vi "NiFPGA Read FIFO - Boolean.vi"(6 "Timeout":u32, 8 "error in (no error)":errorcluster, 9 "Number of Elements":u32, 10 "FIFO":u32, 11 "Session":u32) -> (0 "error out":errorcluster, 1 "Data":bool[](array[boolean]), 3 "Session Out":u32, 4 "Elements Remaining":u32)   [LabVIEW 2010, in "FPGA Interface Wrapper.lvlib"]
doc: "Reads from a FIFO of booleans."
uses:
  <userlib>/_FPGA Interface Advanced Tools/FPGA Interface Wrapper/FPGA Interface Wrapper.lvlib
  NiFpga.dll
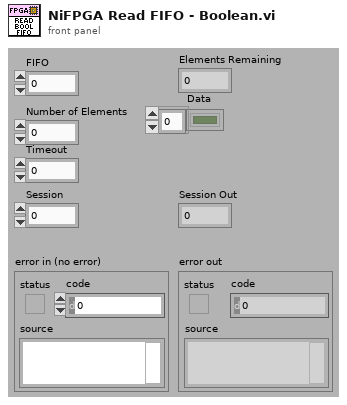
[diagram p1: front panel]
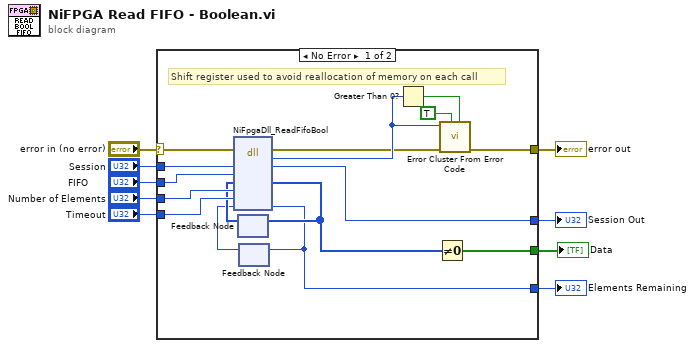
[diagram p0: block diagram]
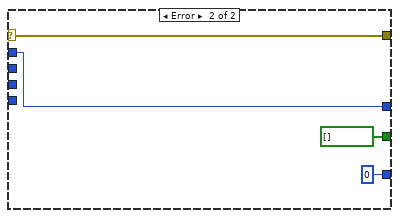
[diagram p2: hidden frame]
diagram:
  n1 = case shown="No Error" "error in (no error)" {
    selector: "error in (no error)" -> [w25 w28]
    tunnel: [w14 w28] -> w8
    tunnel: "Session" -> [w24 w29]
    tunnel: [w23 w29] -> w6
    tunnel: "FIFO" -> [w22 _]
    tunnel: "Number of Elements" -> [w21 _]
    tunnel: "Timeout" -> [w20 _]
    tunnel: [w10 u64 0 ("Elements Remaining")] -> w2
    tunnel: [w19 bool[] []] -> w1
    frame No Error {
      # "Shift register used to avoid reallocation of memory on each call"
      n2 = feedback #1() -> (w12:u8[])  [unwired: 1 in]
      n3 = feedback #2() -> (w11:u64)  [unwired: 1 in]
      n4 = dll-call lib="NiFpga.dll" fn="NiFpgaDll_ReadFifoBool"(error in=w25, "Session"=w24, "FIFO"=w22, "Data"=w12, "Number of Elements"=w21, "Timeout"=w20, "Elements Remaining"=w11) -> (error out=w15:errorcluster, "Status"=w16:i32, "Session"=w23:u32, "Data"=w13:u8[], "Elements Remaining"=w10:u64)  [unwired: 5 in, 1 out]
      n5 = feedback-in #1(w13) -> ()
      n6 = feedback-in #2(w10) -> ()
      n7 = Greater Than 0?(x=w16) -> (x > 0?=w17:bool)
      n8 = Not Equal To 0?(x=w13) -> (x != 0?=w19:bool[])
      n9 = call <vilib>:"Error Cluster From Error Code.vi"("is warning? (False)"=w17, "show call chain? (False)"=TRUE, "error in (no error)"=w15, "error code (0)"=w16) -> ("error out"=w14:errorcluster)  [unwired: 5 in]
    }
    frame Error {
    }
  }
  "error out" <- w8
  "Session Out" <- w6
  "Elements Remaining" <- w2
  "Data" <- w1
